vi "SEARCH PGSQL FOR ITEMS.vi"(11 "REFERENCES":T1) -> ()   [LabVIEW 2019]
uses:
  Controls/References Cluster.ctl
  Controls/Custom Calendar/Custom Calendar.xctl
  <vilib>/addons/database/Auxilliary.llb/DB Tools Cursor Type.ctl
  Controls/Table Data Types/Inventory Data Type.ctl
  Controls/Column Names/Inventory Column Names.ctl
  <vilib>/addons/database/Connection.llb/DB Tools Open Connec (String).vi
  <vilib>/addons/database/Connection.llb/Conn Execute.vi
  <vilib>/addons/database/Recordset.llb/Rec Fetch Recordset Data (R).vi
  <vilib>/addons/database/Recordset.llb/Rec Destroy - Connection.vi
  <vilib>/addons/database/_DB Variant To Data/Database Variant To Data.xnode
  <vilib>/addons/database/NI_Database_API.lvlib
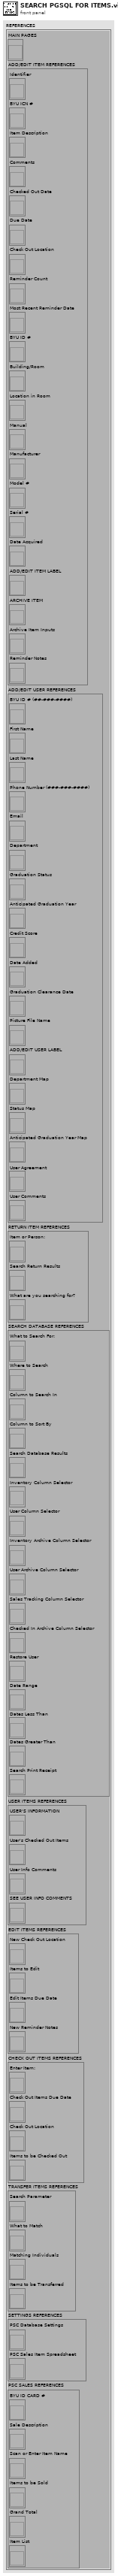
[diagram p1: front panel]
types:
  T1 = typedef "References Cluster.ctl" = cluster{"MAIN PAGES":refnum<vi>, "ADD/EDIT ITEM REFERENCES":cluster{"Identifier":refnum<vi>, "BYU ICN #":refnum<vi>, "Item Description":refnum<vi>, "Comments":refnum<vi>, "Checked Out Date":refnum<vi>, "Due Date":refnum<vi>, "Check Out Location":refnum<vi>, "Reminder Count":refnum<vi>, "Most Recent Reminder Date":refnum<vi>, "BYU ID #":refnum<vi>, "Building/Room":refnum<vi>, "Location in Room":refnum<vi>, "Manual":refnum<vi>, "Manufacturer":refnum<vi>, "Model #":refnum<vi>, "Serial #":refnum<vi>, "Date Acquired":refnum<vi>, "ADD/EDIT ITEM LABEL":refnum<vi>, "ARCHIVE ITEM":refnum<vi>, "Archive Item Inputs":refnum<vi>, "Reminder Notes":refnum<vi>}, "ADD/EDIT USER REFERENCES":cluster{"BYU ID # (##-###-####)":refnum<vi>, "First Name":refnum<vi>, "Last Name":refnum<vi>, "Phone Number (###-###-####)":refnum<vi>, "Email":refnum<vi>, "Department":refnum<vi>, "Graduation Status":refnum<vi>, "Anticipated Graduation Year":refnum<vi>, "Credit Score":refnum<vi>, "Date Added":refnum<vi>, "Graduation Clearance Date":refnum<vi>, "Picture File Name":refnum<vi>, "ADD/EDIT USER LABEL":refnum<vi>, "Department Map":refnum<vi>, "Status Map":refnum<vi>, "Anticipated Graduation Year Map":refnum<vi>, "User Agreement":refnum<vi>, "User Comments":refnum<vi>}, "RETURN ITEM REFERENCES":cluster{"Item or Person:":refnum<vi>, "Search Return Results":refnum<vi>, "What are you searching for?":refnum<vi>}, "SEARCH DATABASE REFERENCES":cluster{"What to Search For:":refnum<vi>, "Where to Search":refnum<vi>, "Column to Search In":refnum<vi>, "Column to Sort By":refnum<vi>, "Search Database Results":refnum<vi>, "Inventory Column Selector":refnum<vi>, "User Column Selector":refnum<vi>, "Inventory Archive Column Selector":refnum<vi>, "User Archive Column Selector":refnum<vi>, "Sales Tracking Column Selector":refnum<vi>, "Checked In Archive Column Selector":refnum<vi>, "Restore User":refnum<vi>, "Date Range":refnum<vi>, "Dates Less Than":refnum<vi>, "Dates Greater Than":refnum<vi>, "Search Print Receipt":refnum<vi>}, "USER ITEMS REFERENCES":cluster{"USER'S INFORMATION":refnum<vi>, "User's Checked Out Items":refnum<vi>, "User Info Comments":refnum<vi>, "SEE USER INFO COMMENTS":refnum<vi>}, "EDIT ITEMS REFERENCES":cluster{"New Check Out Location":refnum<vi>, "Items to Edit":refnum<vi>, "Edit Items Due Date":refnum<vi>, "New Reminder Notes":refnum<vi>}, "CHECK OUT ITEMS REFERENCES":cluster{"Enter Item:":refnum<vi>, "Check Out Items Due Date":refnum<vi>, "Check Out Location":refnum<vi>, "Items to be Checked Out":refnum<vi>}, "TRANSFER ITEMS REFERENCES":cluster{"Search Parameter":refnum<vi>, "What to Match":refnum<vi>, "Matching Individuals":refnum<vi>, "Items to be Transferred":refnum<vi>}, "SETTINGS REFERENCES":cluster{"PSC Database Settings":refnum<vi>, "PSC Sales Item Spreadsheet":refnum<vi>}, "PSC SALES REFERENCES":cluster{"BYU ID CARD #":refnum<vi>, "Sale Description":refnum<vi>, "Scan or Enter Item Name":refnum<vi>, "Items to be Sold":refnum<vi>, "Grand Total":refnum<vi>, "Item List":refnum<vi>}}
  T2 = typedef "Inventory Column Names.ctl" = string[]
  T3 = typedef "Inventory Data Type.ctl" = cluster{"Identifier":string, "BYU ICN #":string, "Item Description":string, "Comments":string, "Checked Out Date":string, "Due Date":string, "Check Out Location":string, "Reminder Count":i32, "Most Recent Reminder Date":string, "BYU ID #":string, "Building/Room":string, "Location in Room":string, "Manual":string, "Manufacturer":string, "Model #":string, "Serial #":string, "Date Acquired":string, "Reminder Notes":string}
  T4 = typedef "NI_Database_API.lvlib/DB Tools Cursor Type.ctl" = enum16{"forward-only", "keyset", "dynamic", "static"}
  T5 = cluster{"Item or Person:":refnum<vi>, "Search Return Results":refnum<vi>, "What are you searching for?":refnum<vi>}
  T6 = typedef "NI_Database_API.lvlib/Conn ObjectReference.ctl" = refnum<k1>
  T7 = typedef "NI_Database_API.lvlib/Rec ObjectReference.ctl" = refnum<k1>
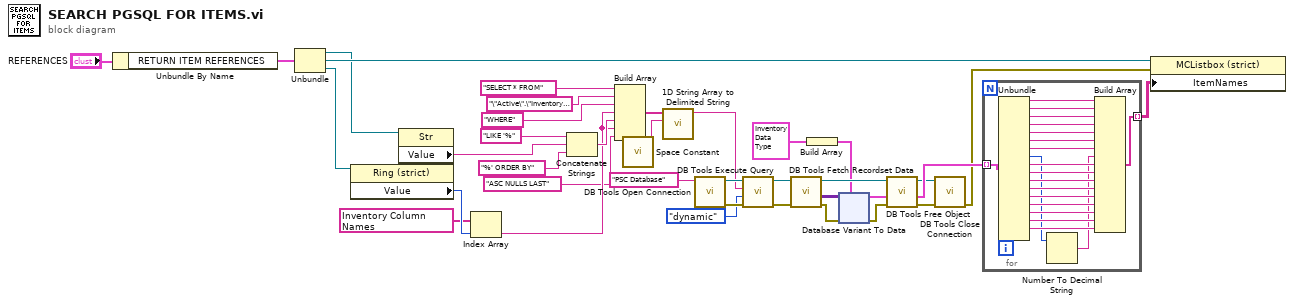
[diagram p0: block diagram]
diagram:
  n1 = Unbundle By Name("REFERENCES") -> ("RETURN ITEM REFERENCES"=w14:T5)
  n2 = Unbundle(w14) -> ("Item or Person:"=w25:refnum<vi>, "Search Return Results"=w26:refnum<vi>, "What are you searching for?"=w24:refnum<vi>)
  n3 = property class="Ring (strict)"(reference=w24) -> ("Value"=w19:u16)  [unwired: 1 in, 2 out]
  n4 = property class="Str"(reference=w25) -> ("Value"=w17:string)  [unwired: 1 in, 2 out]
  n5 = Index Array(array=T2 ["\"Identifier\"", "BYU ICN #", "Item Description", "Comments", "Checked Out Date", "Due Date", "Check Out Location", "Reminder Count", "Most Recent Reminder Date", "BYU ID #", "Building/Room", "Location in Room", "Manual", "Manufacturer", "Model #", "Serial #", "Date Acquired"] ("INVENTORY COLUMN NAMES"), index=w19) -> (element=w5:string)
  n6 = Concatenate Strings("LIKE '%", w17, "%' ORDER BY") -> (w6:string)
  n7 = Build Array("SELECT * FROM" ("SQL query"), "\"Active\".\"Inventory\"", "WHERE", w5, w6, w5, "ASC NULLS LAST") -> (w3:string[])
  n8 = call <vilib>:"Space Constant.vi"() -> ("String"=w2:string)
  n9 = call <vilib>:"1D String Array to Delimited String.vi"("delimiter"=w2, "string array"=w3) -> ("delimited string"=w1:string)  [unwired: 9 in]
  n10 = call-poly <vilib>:"DB Tools Open Connection.vi"("connection information"="PSC Database") -> ("error out"=w36:errorcluster, "connection reference"=w32:T6)  [unwired: 7 in]
  n11 = call-poly <vilib>:"DB Tools Execute Query.vi"("error in (no error)"=w36, "cursor type"=DB_Tools_Cursor_Type."dynamic", "SQL query"=w1, "connection reference"=w32) -> ("error out"=w33:errorcluster, "recordset reference"=w34:T7)  [unwired: 4 in]
  n12 = call-poly <vilib>:"DB Tools Fetch Recordset Data.vi"("error in (no error)"=w33, "recordset reference"=w34) -> ("error out"=w30:errorcluster, "recordset data"=w31:variant[][], "recordset reference out"=w20:T7)  [unwired: 3 in]
  n13 = Build Array(T3 {"Identifier"="", "BYU ICN #"="", "Item Description"="", "Comments"="", "Checked Out Date"="", "Due Date"="", "Check Out Location"="", "Reminder Count"=0, "Most Recent Reminder Date"="", "BYU ID #"="", "Building/Room"="", "Location in Room"="", "Manual"="", "Manufacturer"="", "Model #"="", "Serial #"="", "Date Acquired"="", "Reminder Notes"=""}) -> (w10:T3[])
  n14 = xnode "Database Variant To Data"("database variant"=w31, "error in (no error)"=w30, "type"=w10) -> ("data"=w29:T3[], "error out"=w23:errorcluster)
  n15 = call-poly <vilib>:"DB Tools Free Object.vi"("error in (no error)"=w23, "recordset reference"=w20) -> ("error out"=w21:errorcluster, "connection reference"=w22:T6)  [unwired: 8 in]
  n16 = call <vilib>:"DB Tools Close Connection.vi"("error in (no error)"=w21, "connection reference"=w22) -> ("error out"=w27:errorcluster)  [unwired: 5 in]
  n17 = for {
    tunnel: w29 -> [w56] mode=indexing
    tunnel: [w40] -> w28 mode=indexing
    n18 = Unbundle(w56) -> ("Identifier"=w55:string, "BYU ICN #"=w54:string, "Item Description"=w53:string, "Comments"=w52:string, "Checked Out Date"=w51:string, "Due Date"=w50:string, "Check Out Location"=w49:string, "Reminder Count"=w38:i32, "Most Recent Reminder Date"=w48:string, "BYU ID #"=w47:string, "Building/Room"=w46:string, "Location in Room"=w45:string, "Manual"=w44:string, "Manufacturer"=w43:string, "Model #"=w39:string, "Serial #"=w42:string, "Date Acquired"=w41:string)  [unwired: 1 out]
    n19 = Number To Decimal String(number=w38) -> (decimal integer string=w37:string)  [unwired: 1 in]
    n20 = Build Array(w55, w54, w53, w52, w51, w50, w49, w37, w48, w47, w46, w45, w44, w43, w39, w42, w41) -> (w40:string[])
  }
  n21 = property class="MCListbox (strict)"(reference=w26, error in=w27, "ItemNames"=w28) -> ()  [unwired: 2 out]
